vi "TcA07-003_Serialization.vi"(1 "Input buffer":T3="1", 3 "Invocation info":T2, 5 "error in (no error)":errorcluster, 6 "Add log to result?":bool) -> (16 "Test Data":T1 {"Numeric Measurement" format="%.2f"}, 19 "error out":errorcluster)   [LabVIEW 2020]
doc: "Test case template."
uses:
  Shared/Support_InputBuffer.ctl
  Shared/Support_InvocationInfo.ctl
  Shared/Support_TestData.ctl
  TestClasses/G#SubClass1_class/G#SubClass1.lvclass
  TestClasses/G#BaseAggregator_class/G#BaseAggregator.lvclass
  <vilib>/addons/_AddQ/G#Object/G#Object.lvclass
panel:
  in  "Test name":string="TcA07-003 Serialization"
  out "Test result":bool
  out "Result":string
  # "Verify that serialization and deserialization works."
  # "Sub test case"
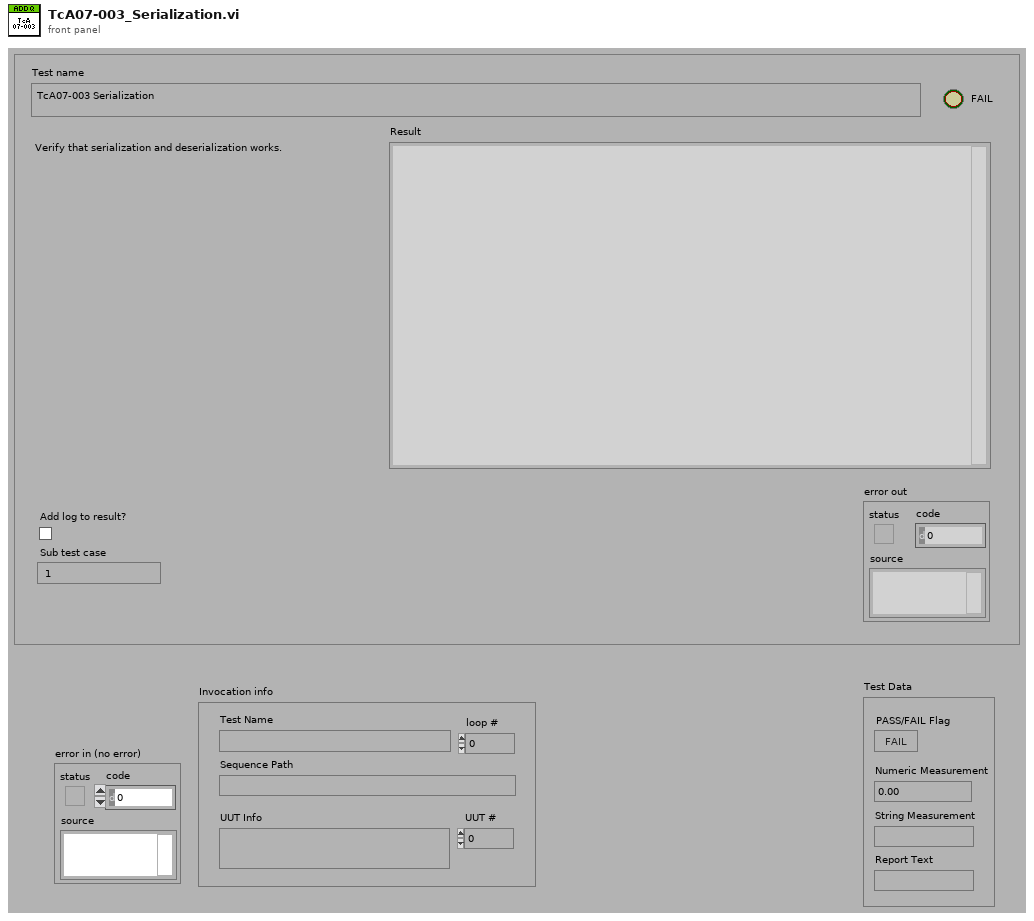
[diagram p1: front panel]
types:
  T1 = typedef "Support_TestData.ctl" = cluster{"PASS/FAIL Flag":bool, "Numeric Measurement":dbl, "String Measurement":string, "Report Text":string}
  T2 = typedef "Support_InvocationInfo.ctl" = cluster{"UUT #":i32, "loop #":i32, "UUT Info":string, "Test Name":string, "Sequence Path":path}
  T3 = typedef "Support_InputBuffer.ctl" = string
  T4 = typedef "Support_ResultType.ctl" = cluster{"Pass":bool, "Comment":string, "MeasurementValue":dbl}
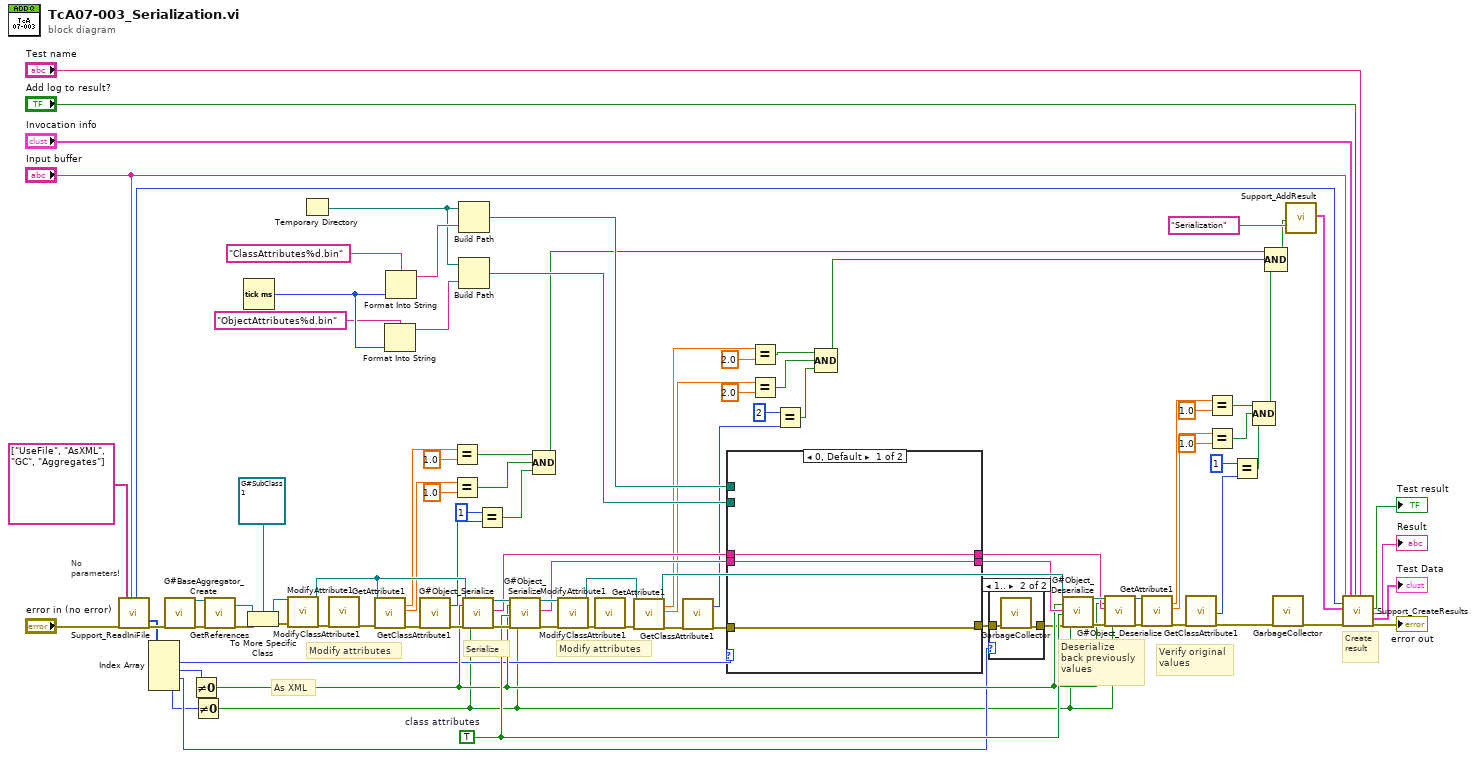
[diagram p0: block diagram]
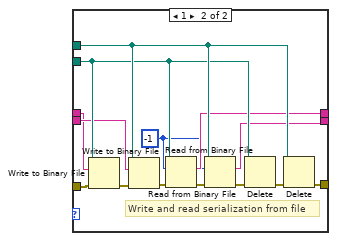
[diagram p3: hidden frame]
diagram:
  w20 = TRUE  # class attributes
  # "As XML"
  # "Verify original\nvalues"
  # "Deserialize\nback previously\nvalues"
  # "Modify attributes"
  # "Serialize"
  # "Modify attributes"
  # "No\nparameters!"
  # "Create\nresult"
  n1 = call "Support_ReadIniFile.vi"("error in (no error)"="error in (no error)", "Parameter names"=string[] ["UseFile", "AsXML", "GC", "Aggregates"], "Sub test case"="Input buffer") -> ("Timer start"=w87:u32, "Parameters as I32"=w8:i32[], "error out"=w17:errorcluster)  [unwired: 9 in, 5 out]
  n2 = Index Array(array=w8) -> (element #1=w6:i32, element #2=w7:i32, element #3=w4:i32, element #4=w2:i32)  [unwired: 4 in]
  n3 = call "G#BaseAggregator_Create.vi"("error in (no error)"=w17) -> ("reference out"=w15:refnum<class "G#BaseAggregator.lvclass">, "error out"=w16:errorcluster)  [unwired: 17 in]
  n4 = Not Equal To 0?(x=w7) -> (x != 0?=w18:bool)
  n5 = Not Equal To 0?(x=w2) -> (x != 0?=w1:bool)
  n6 = call-dynamic "GetReferences.vi"("reference in"=w15, "error in (no error)"=w16) -> ("G#BaseClass1.lvclass"=w12:refnum<class "G#BaseClass1.lvclass">, "error out"=w14:errorcluster)  [unwired: 14 in, 2 out]
  n7 = Tick Count (ms)() -> (millisecond timer value=w58:u32)
  n8 = To More Specific Class(target class=refnum<class "G#SubClass1.lvclass"> refnum ("reference in"), reference=w12, error in=w14) -> (specific class reference=w10:refnum<class "G#SubClass1.lvclass">, error out=w13:errorcluster)
  n9 = call-dynamic "ModifyAttribute1.vi"("reference in"=w10, "error in (no error)"=w13) -> ("reference out"=w79:refnum<class "G#SubClass1.lvclass">, "error out"=w83:errorcluster)  [unwired: 16 in]
  n10 = Temporary Directory() -> (w56:path)
  n11 = call "ModifyClassAttribute1.vi"("error in (no error)"=w83) -> ("error out"=w82:errorcluster)  [unwired: 18 in]
  n12 = call-dynamic "GetAttribute1.vi"("reference in"=w79, "error in (no error)"=w82) -> ("Base class.Numeric"=w51:dbl, "SubAttribute"=w50:dbl, "error out"=w81:errorcluster)  [unwired: 13 in, 2 out]
  n13 = Format Into String(format string="ObjectAttributes%d.bin", w58) -> (resulting string=w55:string)  [unwired: 2 in, 1 out]
  n14 = Format Into String(format string="ClassAttributes%d.bin", w58) -> (resulting string=w57:string)  [unwired: 2 in, 1 out]
  n15 = call "GetClassAttribute1.vi"("error in (no error)"=w81) -> ("Int"=w47:i32, "error out"=w80:errorcluster)  [unwired: 15 in, 2 out]
  n16 = Equal?(x=w51, y=1.0) -> (x = y?=w39:bool)
  n17 = Equal?(x=w50, y=1.0) -> (x = y?=w38:bool)
  n18 = Build Path(base path=w56, name or relative path=w57) -> (appended path=w53:path)
  n19 = Build Path(base path=w56, name or relative path=w55) -> (appended path=w52:path)
  n20 = call-dynamic "G#Object_Serialize.vi"("reference in"=w79, "as xml (F)"=w18, "error in (no error)"=w80, "include aggregates (T)"=w1) -> ("reference out"=w71:refnum<class "G#SubClass1.lvclass">, "serialized object"=w66:string, "error out"=w72:errorcluster)  [unwired: 12 in, 1 out]
  n21 = Equal?(x=1, y=w47) -> (x = y?=w37:bool)
  n22 = call-dynamic "G#Object_Serialize.vi"("reference in"=w71, "as xml (F)"=w18, "class attributes (F)"=w20, "error in (no error)"=w72, "include aggregates (T)"=w1) -> ("reference out"=w69:refnum<class "G#SubClass1.lvclass">, "serialized object"=w65:string, "error out"=w70:errorcluster)  [unwired: 11 in, 1 out]
  n23 = Compound Arithmetic op=AND(w39, w38, w37) -> (w22:bool)
  n24 = call-dynamic "ModifyAttribute1.vi"("reference in"=w69, "error in (no error)"=w70) -> ("reference out"=w74:refnum<class "G#SubClass1.lvclass">, "error out"=w78:errorcluster)  [unwired: 16 in]
  n25 = call "ModifyClassAttribute1.vi"("error in (no error)"=w78) -> ("error out"=w77:errorcluster)  [unwired: 18 in]
  n26 = call-dynamic "GetAttribute1.vi"("reference in"=w74, "error in (no error)"=w77) -> ("reference out"=w73:refnum<class "G#SubClass1.lvclass">, "Base class.Numeric"=w42:dbl, "SubAttribute"=w41:dbl, "error out"=w76:errorcluster)  [unwired: 13 in, 1 out]
  n27 = call "GetClassAttribute1.vi"("error in (no error)"=w76) -> ("Int"=w40:i32, "error out"=w75:errorcluster)  [unwired: 15 in, 2 out]
  n28 = case shown="0, Default" w6 {
    tunnel: w75 -> [w99 w113]
    tunnel: [w99 w106] -> w5
    tunnel: w66 -> [w97 w102]
    tunnel: w65 -> [w98 w104]
    tunnel: [w98 w103] -> w64
    tunnel: [w97 w101] -> w63
    tunnel: w53 -> [_ w108]
    tunnel: w52 -> [_ w105]
    frame 0, Default {
    }
    frame 1 {
      w100 = -1 ("count (1)")
      # "Write and read serialization from file"
      n29 = Write to Binary File(file (use dialog)=w105, data=w102, error in=w113) -> (error out=w112:errorcluster)  [unwired: 3 in, 2 out]
      n30 = Write to Binary File(file (use dialog)=w108, data=w104, error in=w112) -> (error out=w111:errorcluster)  [unwired: 3 in, 2 out]
      n31 = Read from Binary File(8:w111, 10:w100, 11:w105) -> (0:w110:errorcluster, 2:w101:string)  [unwired: 3 in, 2 out]
      n32 = Read from Binary File(8:w110, 10:w100, 11:w108) -> (0:w109:errorcluster, 2:w103:string)  [unwired: 3 in, 2 out]
      n33 = Delete(path (use dialog)=w105, error in=w109) -> (error out=w107:errorcluster)  [unwired: 3 in, 2 out]
      n34 = Delete(path (use dialog)=w108, error in=w107) -> (error out=w106:errorcluster)  [unwired: 3 in, 2 out]
    }
  }
  n35 = Equal?(x=w42, y=2.0) -> (x = y?=w36:bool)
  n36 = Equal?(x=w41, y=2.0) -> (x = y?=w35:bool)
  n37 = Equal?(x=2, y=w40) -> (x = y?=w34:bool)
  n38 = Compound Arithmetic op=AND(w36, w35, w34) -> (w23:bool)
  n39 = case shown="1.." w4 {
    tunnel: w5 -> [w114 w116]
    tunnel: [w114 w115] -> w3
    frame 0, Default {
    }
    frame 1.. {
      n40 = call <vilib>:"GarbageCollector.vi"("error in (no error)"=w116) -> ("error out"=w115:errorcluster)  [unwired: 16 in, 2 out]
    }
  }
  n41 = call-dynamic "G#Object_Deserialize.vi"("reference in"=w73, "as xml (F)"=w18, "serialized object"=w64, "class attributes (F)"=w20, "error in (no error)"=w3, "include aggregates (T)"=w1) -> ("reference out"=w68:refnum<class "G#SubClass1.lvclass">, "error out"=w67:errorcluster)  [unwired: 11 in, 1 out]
  n42 = call-dynamic "G#Object_Deserialize.vi"("reference in"=w68, "as xml (F)"=w18, "serialized object"=w63, "error in (no error)"=w67, "include aggregates (T)"=w1) -> ("reference out"=w60:refnum<class "G#SubClass1.lvclass">, "error out"=w62:errorcluster)  [unwired: 12 in, 1 out]
  n43 = call-dynamic "GetAttribute1.vi"("reference in"=w60, "error in (no error)"=w62) -> ("Base class.Numeric"=w27:dbl, "SubAttribute"=w26:dbl, "error out"=w61:errorcluster)  [unwired: 13 in, 2 out]
  n44 = call "GetClassAttribute1.vi"("error in (no error)"=w61) -> ("SubClassIntAttribute"=w25:i32, "error out"=w9:errorcluster)  [unwired: 15 in, 2 out]
  n45 = Equal?(x=w27, y=1.0) -> (x = y?=w31:bool)
  n46 = Equal?(x=w26, y=1.0) -> (x = y?=w32:bool)
  n47 = Equal?(x=1, y=w25) -> (x = y?=w33:bool)
  n48 = Compound Arithmetic op=AND(w31, w32, w33) -> (w24:bool)
  n49 = Compound Arithmetic op=AND(w22, w23, w24) -> (w21:bool)
  n50 = call <vilib>:"GarbageCollector.vi"("error in (no error)"=w9) -> ("error out"=w86:errorcluster)  [unwired: 16 in, 2 out]
  n51 = call "Support_AddResult.vi"("Pass"=w21, "Comment"="Serialization") -> ("Results out"=w85:T4[])  [unwired: 17 in]
  n52 = call "Support_CreateResults.vi"("Sub test case"="Input buffer", "Timer start"=w87, "Results"=w85, "error in (no error)"=w86, "Invocation info"="Invocation info", "Add log to result?"="Add log to result?", "Test name"="Test name") -> ("Pass/fail flag"=→"Test result":bool, "Result"=→"Result":string, "Test Data"=→"Test Data":T1, "error out"=→"error out":errorcluster)  [unwired: 9 in]
